vi "Configure Clock Recovery Method Edge.vi"(8 "error in (no error)":errorcluster, 10 "Edge Type (2: Both)":i32(ring)=2 items=["Rising", "Falling", "Both"], 11 "VISA resource name":refnum<visa-resource-name>) -> (0 "error out":errorcluster, 3 "VISA resource name out":refnum<visa-resource-name>)   [LabVIEW 2020, in "Agilent 90000 Series.lvlib"]
doc: "Configures which edge(s) of the data are used to recover a clock.\n\n<b>Note:</b>\nThis VI is new in firmware version 4.30."
uses:
  Agilent 90000 Series.lvlib
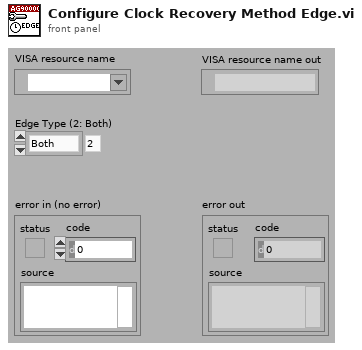
[diagram p1: front panel]
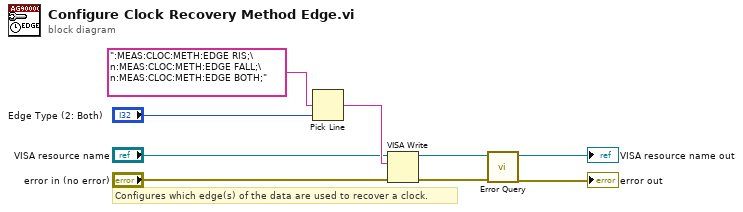
[diagram p0: block diagram]
diagram:
  # "Configures which edge(s) of the data are used to recover a clock."
  n1 = Pick Line(multi-line string=":MEAS:CLOC:METH:EDGE RIS;\n:MEAS:CLOC:METH:EDGE FALL;\n:MEAS:CLOC:METH:EDGE BOTH;", line index="Edge Type (2: Both)") -> (output string=w7:string)  [unwired: 1 in]
  n2 = VISA Write(VISA resource name="VISA resource name", write buffer=w7, error in (no error)="error in (no error)") -> (VISA resource name out=w4:refnum<visa-resource-name>, error out=w3:errorcluster)  [unwired: 1 out]
  n3 = call "Error Query.vi"("error in (no error)"=w3, "VISA resource name"=w4) -> ("error out"=→"error out":errorcluster, "VISA resource name out"=→"VISA resource name out":refnum<visa-resource-name>)  [unwired: 6 in, 2 out]
